vi "Sensors.vi"() -> ()   [LabVIEW 2023]
panel:
  out "humidity-indoor":u8
  out "temp-indoor":u8
  out "roof-window-open":bool
  out "light-gain":dbl
  out "temp-outdoor":dbl format="%#_3g"
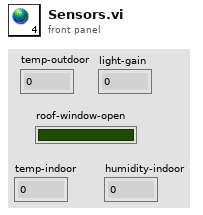
[diagram p1: front panel]
diagram:
